vi "test Acyclic Loopback.vi"(8 "error in":errorcluster, 11 "TestCase in":refnum<class "Single Board Loopback.lvclass">) -> (0 "error out":errorcluster, 3 "TestCase out":refnum<class "Single Board Loopback.lvclass">)   [LabVIEW 2020, in "Single Board Loopback.lvclass"]
uses:
  Single Board Loopback.lvclass
  <vilib>/addons/_JKI Toolkits/VI Tester/TestCase.llb/TestCase.lvclass
  <vilib>/NI VeriStand/Execution/Workspace/NI_VS Workspace ExecutionAPI.lvlib
  <vilib>/NI/VeriStand Custom Device Testing Tools/VeriStandTestUtilities/VeriStandTestUtilities.lvlib
  <vilib>/NI VeriStand/Execution/Workspace/NI VeriStand - Set Multiple Channel Values.vi
  <vilib>/numeric/Random Number (Range) U64.vi
  C:/Users/nitest/Desktop/Git 2020/niveristand-custom-device-testing-tools/VeriStandTestCase/VeriStandTestCase.lvclass
  C:/Program Files (x86)/National Instruments/LabVIEW 2020/vi.lib/addons/_JKI Toolkits/VI Tester/TestCase.llb/TestCase.lvclass
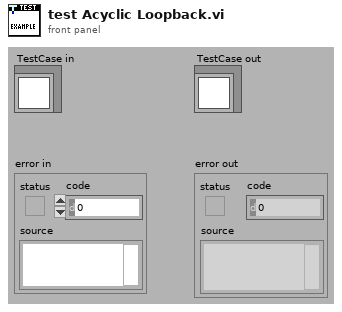
[diagram p1: front panel]
types:
  T1 = typedef "NI_VS Workspace ExecutionAPI.lvlib/WorkspaceAPI.ctl" = refnum<k24>
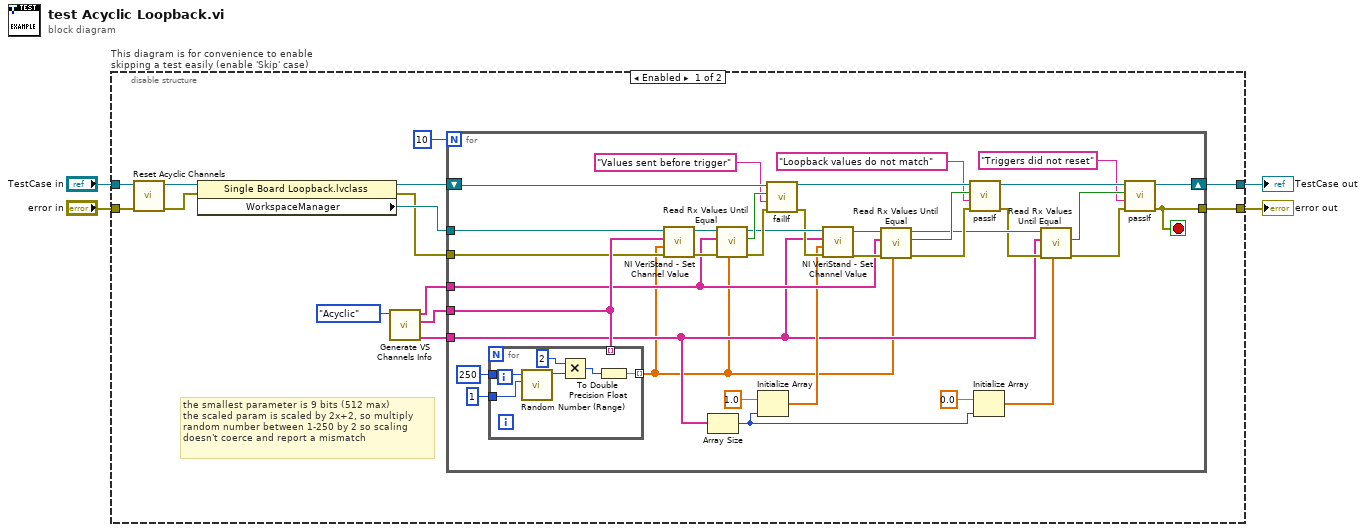
[diagram p0: block diagram]
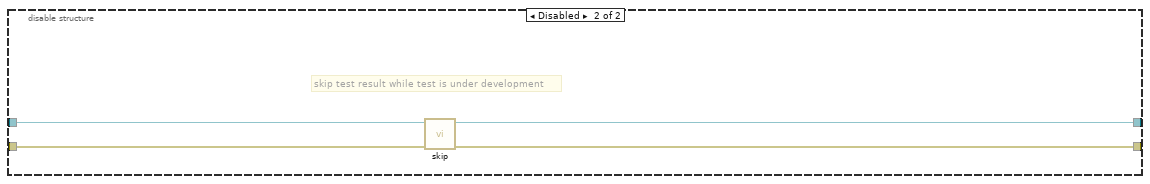
[diagram p2: hidden frame]
diagram:
  n1 = disable-structure "This diagram is for convenience to enable skipping a test easily (enable 'Skip' case)" shown="Enabled" {
    disable-tunnel: "TestCase in" -> [w6 w63]
    disable-tunnel: [w12 w61] -> w1
    disable-tunnel: [w11 w62] -> w3
    disable-tunnel: "error in" -> [w13 w60]
    frame Enabled {
      # "the smallest parameter is 9 bits (512 max)\nthe scaled param is scaled by 2x+2, so multiply \nrandom number between 1-250 by 2 so scaling\ndoesn't coerce and report a mismatch"
      n2 = call "Reset Acyclic Channels.vi"("error in (no error)"=w13, "reference in"=w6) -> ("error out"=w7:errorcluster, "reference out"=w5:refnum<class "Single Board Loopback.lvclass">)  [unwired: 8 in]
      n3 = property class="Single Board Loopback.lvclass"(reference=w5, error in=w7) -> (reference out=w15:refnum<class "Single Board Loopback.lvclass">, error out=w16:errorcluster, "WorkspaceManager"=w17:T1)
      n4 = call "Generate VS Channels Info.vi"("Transfer Type"=enum16{"Acyclic", "Scheduled"}."Acyclic") -> ("Tx Trigger Channels Array"=w9:string[], "Tx Channels Array"=w10:string[], "Rx Channels Array"=w18:string[])  [unwired: 6 in, 2 out]
      n5 = for {
        N: 10 -> [_]
        tunnel: w18 -> [w39]
        tunnel: w17 -> [w51]
        tunnel: w16 -> [w44]
        tunnel: w10 -> [w50]
        shift-right: [w33] -> w12
        shift-left: w15 -> [w46]
        tunnel: [w35] -> w11
        tunnel: w9 -> [w23]
        stop <- w35 stop-if-true
        n6 = for {
          tunnel: [w58] -> w19 mode=indexing
          tunnel: u64 250 ("upper bound (100)") -> [w57]
          tunnel: u64 1 ("upper bound (100)") -> [w56]
          tunnel: w50 -> [_] mode=indexing
          n7 = call-poly <vilib>:"Random Number (Range).vi"("lower bound (0)"=w56, "upper bound (100)"=w57) -> ("number"=w59:u64)  [unwired: 9 in]
          n8 = Multiply(x=u64 2, y=w59) -> (x*y=w55:u64)
          n9 = To Double Precision Float(number=w55) -> (double precision float=w58:dbl)
        }
        n10 = call-poly <vilib>:"NI VeriStand - Set Channel Value.vi"("error in (no error)"=w44, "Values"=w19, "Channels"=w50, "WorkspaceManager in"=w51) -> ("error out"=w47:errorcluster, "WorkspaceManager out"=w49:T1)  [unwired: 6 in]
        n11 = Array Size(array=w23) -> (size(s)=w20:i32)
        n12 = call <vilib>:"Read Rx Values Until Equal.vi"("expected values"=w19, "error in"=w47, "Rx aliases"=w39, "workspace manager in"=w49) -> ("error out"=w48:errorcluster, "values equal expected"=w45:bool, "workspace manager out"=w43:T1)  [unwired: 5 in]
        n13 = Initialize Array(1.0, w20) -> (w24:dbl[])
        n14 = call-dynamic "failIf.vi"("error in (no error)"=w48, "message (\"\")"="Values sent before trigger" ("message (\"\")"), "fail"=w45, "TestCase in"=w46) -> ("error out"=w42:errorcluster, "TestCase out"=w36:refnum<class "Single Board Loopback.lvclass">)  [unwired: 6 in]
        n15 = call-poly <vilib>:"NI VeriStand - Set Channel Value.vi"("error in (no error)"=w42, "Values"=w24, "Channels"=w23, "WorkspaceManager in"=w43) -> ("error out"=w40:errorcluster, "WorkspaceManager out"=w41:T1)  [unwired: 6 in]
        n16 = call <vilib>:"Read Rx Values Until Equal.vi"("expected values"=w19, "error in"=w40, "Rx aliases"=w39, "workspace manager in"=w41) -> ("error out"=w37:errorcluster, "values equal expected"=w38:bool, "workspace manager out"=w31:T1)  [unwired: 5 in]
        n17 = call-dynamic "passIf.vi"("error in (no error)"=w37, "message (\"\")"="Loopback values do not match" ("message (\"\")"), "pass"=w38, "TestCase in"=w36) -> ("error out"=w30:errorcluster, "TestCase out"=w34:refnum<class "Single Board Loopback.lvclass">)  [unwired: 6 in]
        n18 = Initialize Array(0.0, w20) -> (w21:dbl[])
        n19 = call <vilib>:"Read Rx Values Until Equal.vi"("expected values"=w21, "error in"=w30, "Rx aliases"=w23, "workspace manager in"=w31) -> ("error out"=w29:errorcluster, "values equal expected"=w32:bool)  [unwired: 5 in, 1 out]
        n20 = call-dynamic "passIf.vi"("error in (no error)"=w29, "message (\"\")"="Triggers did not reset" ("message (\"\")"), "pass"=w32, "TestCase in"=w34) -> ("error out"=w35:errorcluster, "TestCase out"=w33:refnum<class "Single Board Loopback.lvclass">)  [unwired: 6 in]
      }
    }
    frame Disabled {
      # "skip test result while test is under development"
      n21 = call <vilib>:"skip.vi"("error in (no error)"=w60, "TestCase in"=w63) -> ("error out"=w62:errorcluster, "TestCase out"=w61:refnum<class "Single Board Loopback.lvclass">)  [unwired: 8 in]
    }
  }
  "error out" <- w3
  "TestCase out" <- w1
